vi "Test Menu Module API.vi"() -> ()   [LabVIEW 2019]
doc: "Menu Module API Tester."
uses:
  Utility/Controls/Menu_Configuration.ctl
  Menu Module.lvlib
panel:
  in  "Menu Type":enum16{"Root", "Sub", "Child"}(ring)
  out "selected Option":string
  in  "Position":cluster{"Top":i16, "Left":i16}
  in  "Resize the Panel":bool
  in  "Menu_Configuration":T1={"Button_Label_Color"=0, "Button_Color_On"=13762511, "Button_Color_Off"=13762511, "Panel_Color"=13762511, "Extend_Sub_Menu_Icon"=path "C:/Users/SyncSols-4/Desktop/Icon/add-icon.png", "Root_Menu_Data"=[{"Button_Icon"=path "C:/Users/SyncSols-4/Desktop/Icon/Accept-icon.png", "Button_Label"="Test", "Sub_Menu_Data"=[{"Button_Icon"=path "C:/Users/SyncSols-4/Desktop/Icon/floppy-icon.png", "Button_Label"="Save", "Child_Menu_Data"=[]}, {"Button_Icon"=path "C:/Users/SyncSols-4/Desktop/Icon/folder-icon1.png", "Button_Label"="Folder", "Child_Menu_Data"=[]}, {"Button_Icon"=path "C:/Users/SyncSols-4/Desktop/Icon/delete-icon.png", "Button_Label"="Delete", "Child_Menu_Data"=[{"Button_Icon"=path "C:/Users/SyncSols-4/Desktop/Icon/add-icon.png", "Button_Label"="Add"}, {"Button_Icon"=path "C:/Users/SyncSols-4/Desktop/Icon/Stop-red-icon.png", "Button_Label"="Stop"}]}]}, {"Button_Icon"=path "C:/Users/SyncSols-4/Desktop/Icon/add-key-icon.png", "Button_Label"="Key", "Sub_Menu_Data"=[]}, {"Button_Icon"=path "C:/Users/SyncSols-4/Desktop/Icon/Categories-preferences-system-icon.png", "Button_Label"="Setting", "Sub_Menu_Data"=[]}]}
  in  "Init Menu":bool
  in  "Run as Singleton?":bool
  in  "Show Block Diagram":bool
  in  "Refresh Modules":bool
  out "Active Modules":string[](array[string])
  in  "Stop Module":bool
  in  "Select Module":i32(ring)=-1 caption="Select Module\nTo send Request to" items=["All"=-1]
  in  "Run New Module":bool
  in  "Hide Module Panel":bool
  in  "Show Module Panel":bool
  out "Status":string
  # "This VI tests the API for the Module."
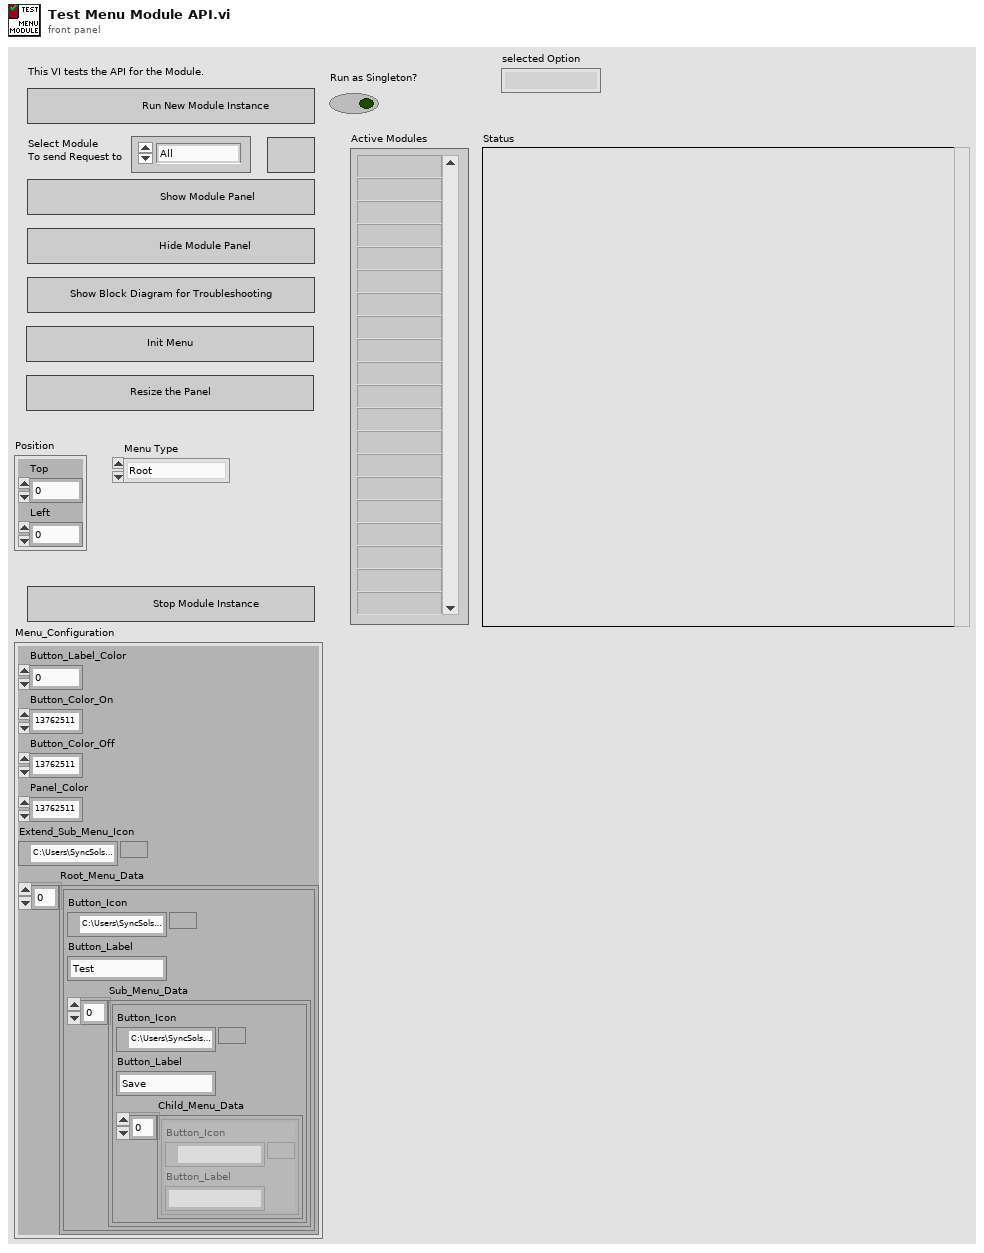
[diagram p1: front panel]
types:
  T1 = typedef "Menu_Configuration.ctl" = cluster{"Button_Label_Color":u32, "Button_Color_On":u32, "Button_Color_Off":u32, "Panel_Color":u32, "Extend_Sub_Menu_Icon":path, "Root_Menu_Data":cluster{"Button_Icon":path, "Button_Label":string, "Sub_Menu_Data":cluster{"Button_Icon":path, "Button_Label":string, "Child_Menu_Data":cluster{"Button_Icon":path, "Button_Label":string}[]}[]}[]}
  T2 = typedef "Menu Module.lvlib/Broadcast Events--cluster.ctl" = cluster{"Module Did Init":refnum<user-event>, "Status Updated":refnum<user-event>, "Error Reported":refnum<user-event>, "Module Did Stop":refnum<user-event>, "Update Module Execution Status":refnum<user-event>, "Button Pressed":refnum<user-event>}
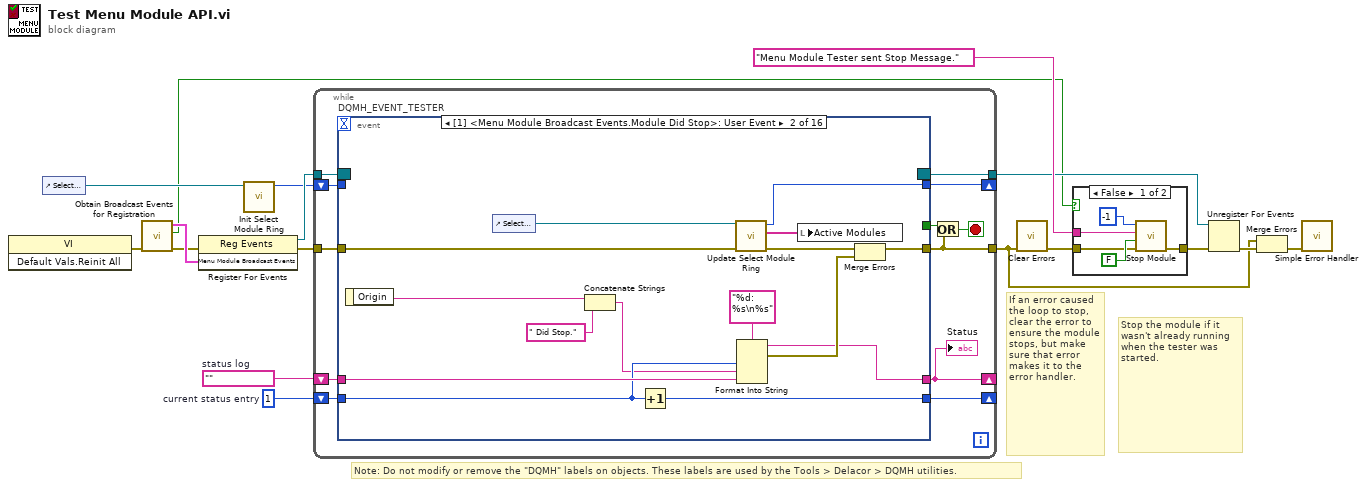
[diagram p0: block diagram]
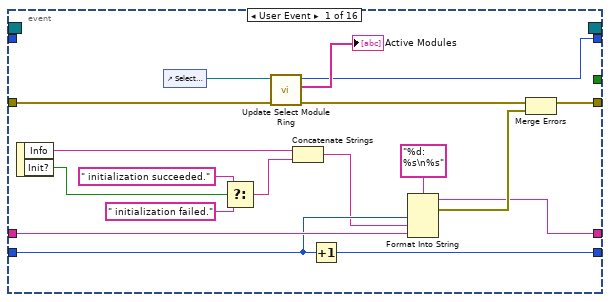
[diagram p3: hidden frame]
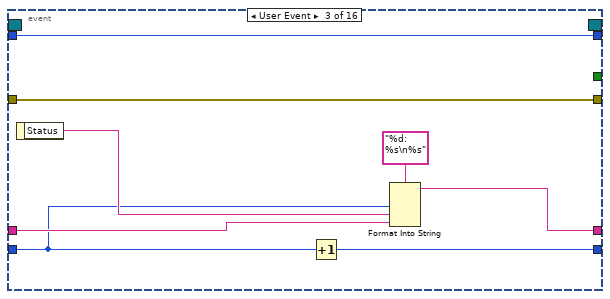
[diagram p4: hidden frame]
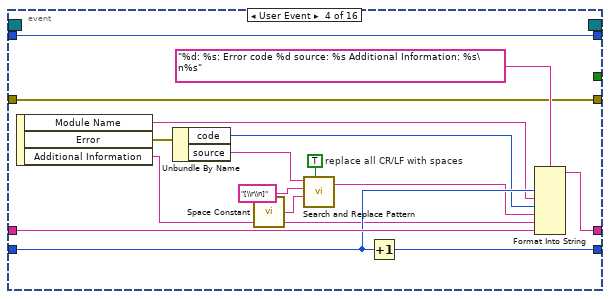
[diagram p5: hidden frame]
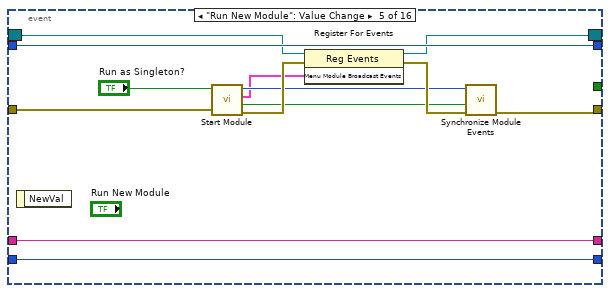
[diagram p6: hidden frame]
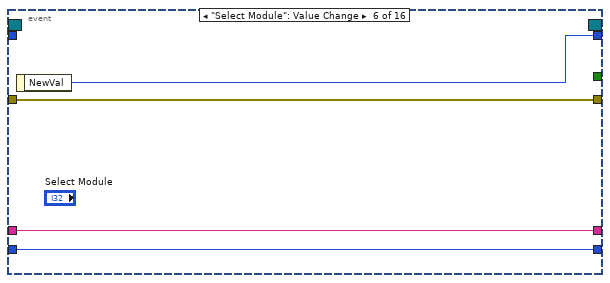
[diagram p7: hidden frame]
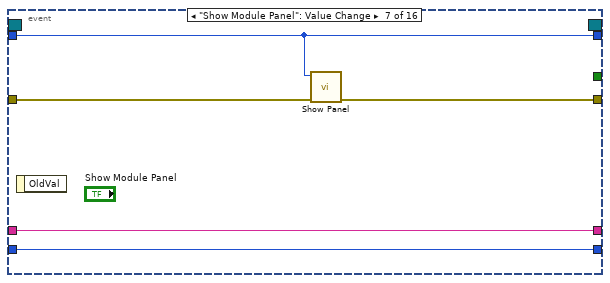
[diagram p8: hidden frame]
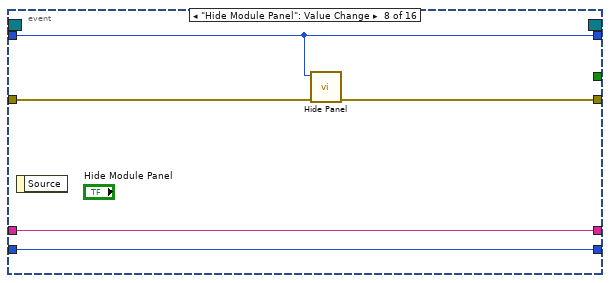
[diagram p9: hidden frame]
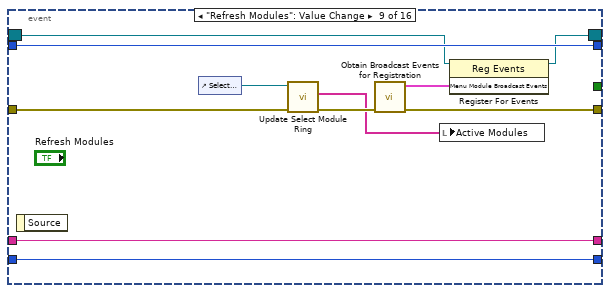
[diagram p10: hidden frame]
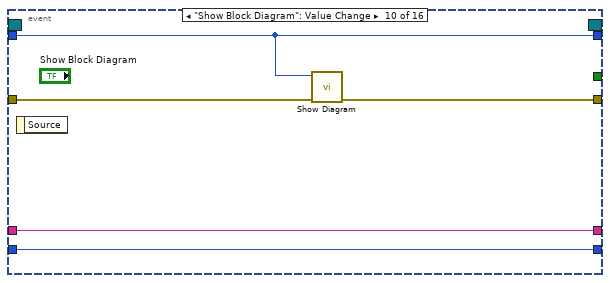
[diagram p11: hidden frame]
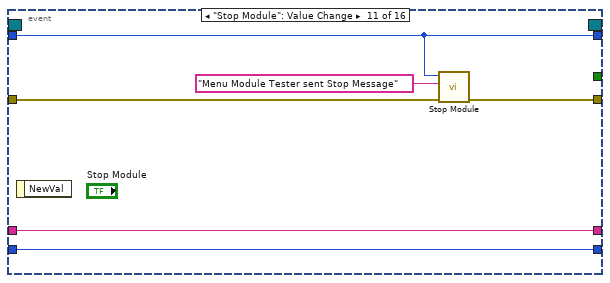
[diagram p12: hidden frame]
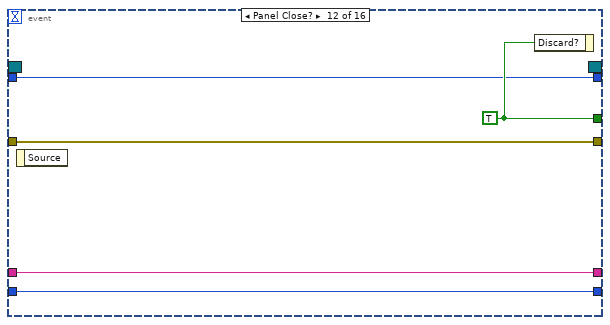
[diagram p13: hidden frame]
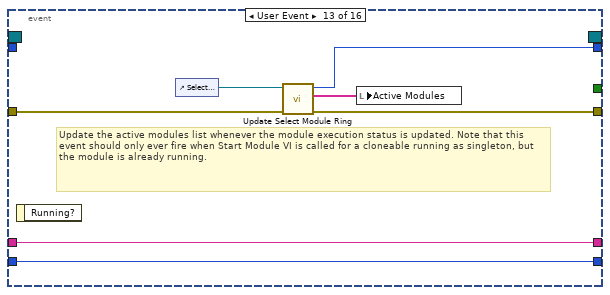
[diagram p14: hidden frame]
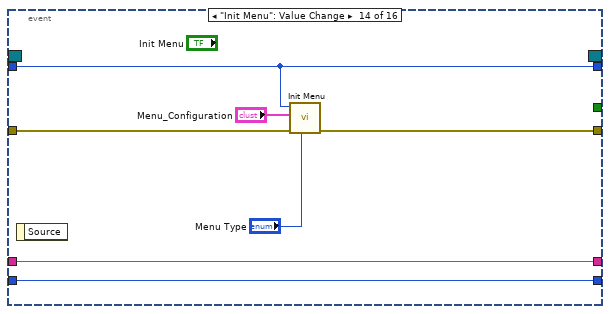
[diagram p15: hidden frame]
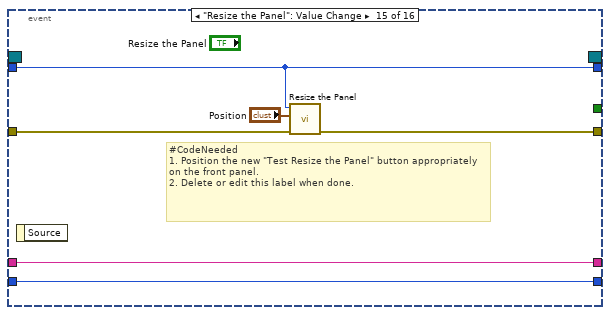
[diagram p16: hidden frame]
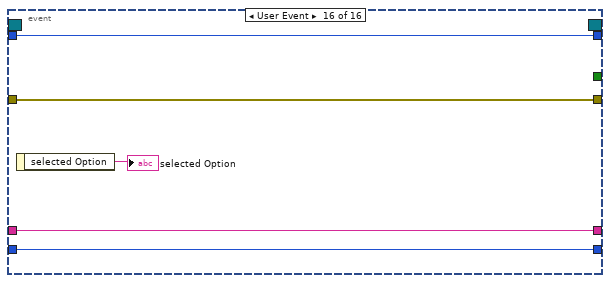
[diagram p17: hidden frame]
diagram:
  w13 = 1  # current status entry
  w14 = ""  # status log
  # "Stop the module if it wasn't already running when the tester was started."
  # "If an error caused the loop to stop, clear the error to ensure the module stops, but make sure that error makes it to the error handler."
  # "Note: Do not modify or remove the \"DQMH\" labels on objects. These labels are used by the Tools > Delacor > DQMH utilities."
  n1 = invoke class="VI" method="Default Vals.Reinit All"() -> (error out=w3:errorcluster)  [unwired: 3 in, 2 out]
  n2 = control-ref of="Select Module"() -> (w11:refnum<vi>)
  n3 = call "Obtain Broadcast Events for Registration.vi"("error in (no error)"=w3) -> ("error out"=w2:errorcluster, "Already running?"=w1:bool, "Menu Module Broadcast Events"=w10:T2)  [unwired: 8 in]
  n4 = register-events(error in=w2, w10) -> (reference out=w17:refnum<event-registration>, error out=w9:errorcluster)  [unwired: 1 in]
  n5 = call "Init Select Module Ring.vi"("Select Module Ring Ref"=w11) -> ("Value for All Modules"=w12:i32)  [unwired: 8 in, 2 out]
  n6 = while {
    tunnel: w17 -> [w29]
    tunnel: [w18] -> w4
    tunnel: w9 -> [w27]
    shift-right: [w23] -> _
    shift-left: w14 -> [w25]
    shift-right: [w24] -> _
    shift-left: w13 -> [w26]
    shift-right: [w20] -> _
    shift-left: w12 -> [w21]
    tunnel: [w19] -> w7
    stop <- w22 stop-if-true
    n7 = event "DQMH_EVENT_TESTER" shown="[1] <Menu Module Broadcast Events.Module Did Stop>: User Event" {
      selector: w29 -> [_ _ _ _ w93 _ _ _ w119 _ _ _ _ _ _ _]
      dyn-events: [_ _ _ _ w92 _ _ _ w118 _ _ _ _ _ _ _] -> w19
      timeout: _ -> [_ _ _ _ _ _ _ _ _ _ _ _ _ _ _ _]
      tunnel: [_ _ _ _ _ _ _ _ _ _ _ w140 _ _ _ _] -> w28
      tunnel: [w37 w54 w70 w76 w91 w103 w107 w112 w115 w126 w131 w139 w143 w151 w157 w165] -> w18
      tunnel: w27 -> [w39 w56 w70 w76 w94 w103 w108 w113 w120 w129 w132 w139 w144 w154 w160 w165]
      tunnel: w26 -> [w44 w59 w63 w82 w96 w101 w105 w110 w123 w127 w134 w137 w146 w152 w158 w163]
      tunnel: w25 -> [w45 w60 w66 w84 w97 w102 w106 w111 w124 w128 w135 w138 w147 w153 w159 w164]
      tunnel: [w42 w57 w67 w79 w97 w102 w106 w111 w124 w128 w135 w138 w147 w153 w159 w164] -> w23
      tunnel: [w43 w58 w69 w85 w96 w101 w105 w110 w123 w127 w134 w137 w146 w152 w158 w163] -> w24
      tunnel: w21 -> [_ _ w64 w86 w95 _ w104 w109 w122 w125 w133 w136 _ w150 w156 w162]
      tunnel: [w34 w51 w64 w86 w95 w100 w104 w109 w122 w125 w133 w136 w142 w150 w156 w162] -> w20
      event User Event {
        n8 = event-data() -> ("Info"=w41:string, "Init?"=w31:bool)  [unwired: 1 in]
        n9 = control-ref of="Select Module"() -> (w36:refnum<vi>)
        n10 = Select(t=" initialization succeeded.", s=w31, f=" initialization failed.") -> (s? t:f=w30:string)
        n11 = call "Update Select Module Ring.vi"("error in (no error)"=w39, "Select Module Ring Ref"=w36) -> ("error out"=w38:errorcluster, "Active Modules (Array)"=→"Active Modules":string[], "New Module Ring Value"=w34:i32)  [unwired: 7 in]
        n12 = Concatenate Strings(w41, w30) -> (w40:string)
        n13 = Increment(x=w44) -> (x+1=w43:i32)
        n14 = Format Into String(format string="%d: %s\n%s", w44, w40, w45) -> (resulting string=w42:string, error out=w47:errorcluster)  [unwired: 2 in]
        n15 = Merge Errors(w38, w47) -> (w37:errorcluster)
      }
      event User Event {
        n16 = event-data() -> ("Origin"=w49:string)  [unwired: 1 in]
        n17 = control-ref of="Select Module"() -> (w53:refnum<vi>)
        n18 = Concatenate Strings(w49, " Did Stop.") -> (w48:string)
        n19 = Increment(x=w59) -> (x+1=w58:i32)
        n20 = call "Update Select Module Ring.vi"("error in (no error)"=w56, "Select Module Ring Ref"=w53) -> ("error out"=w55:errorcluster, "Active Modules (Array)"=w52:string[], "New Module Ring Value"=w51:i32)  [unwired: 7 in]
        n21 = Format Into String(format string="%d: %s\n%s", w59, w48, w60) -> (resulting string=w57:string, error out=w62:errorcluster)  [unwired: 2 in]
        n22 = local write "Active Modules"(w52) -> ()
        n23 = Merge Errors(w55, w62) -> (w54:errorcluster)
      }
      event User Event {
        n24 = event-data() -> ("Status"=w65:string)  [unwired: 1 in]
        n25 = Increment(x=w63) -> (x+1=w69:i32)
        n26 = Format Into String(format string="%d: %s\n%s", w63, w65, w66) -> (resulting string=w67:string)  [unwired: 2 in, 1 out]
      }
      event User Event {
        w80 = TRUE  # replace all CR/LF with spaces
        n27 = event-data() -> ("Module Name"=w74:string, "Error"=w73:errorcluster, "Additional Information"=w71:string)  [unwired: 1 in]
        n28 = Unbundle By Name(w73) -> ("code"=w75:i32, "source"=w77:string)
        n29 = call <vilib>:"Space Constant.vi"() -> ("String"=w81:string)
        n30 = call <vilib>:"Search and Replace Pattern.vi"("string"=w77, "regular expression (\"\")"="[\\r\\n]" ("regular expression (\"\")"), "replace string (\"\")"=w81, "replace all? (F)"=w80) -> ("result string"=w78:string)  [unwired: 1 in, 1 out]
        n31 = Increment(x=w82) -> (x+1=w85:i32)
        n32 = Format Into String(format string="%d: %s: Error code %d source: %s Additional Information: %s\n%s", w82, w74, w75, w78, w71, w84) -> (resulting string=w79:string)  [unwired: 2 in, 1 out]
      }
      event "Run New Module": Value Change {
        n33 = event-data() -> ()  [unwired: 1 in, 1 out]
        n34 = call "Start Module.vi"("error in (no error)"=w94, "Run as Singleton? (F)"="Run as Singleton?") -> ("error out"=w98:errorcluster, "Wait for Event Sync?"=w89:bool, "Menu Module Broadcast Events"=w88:T2, "Module ID"=w90:i32)  [unwired: 6 in]
        n35 = register-events(reference=w93, error in=w98, w88) -> (reference out=w92:refnum<event-registration>, error out=w99:errorcluster)
        n36 = call "Synchronize Module Events.vi"("error in (no error)"=w99, "Wait for Event Sync?"=w89, "Module ID"=w90) -> ("error out"=w91:errorcluster)  [unwired: 7 in, 1 out]
      }
      event "Select Module": Value Change {
        n37 = event-data() -> ("NewVal"=w100:i32)  [unwired: 1 in]
      }
      event "Show Module Panel": Value Change {
        n38 = event-data() -> ()  [unwired: 1 in, 1 out]
        n39 = call "Show Panel.vi"("error in (no error)"=w108, "Module ID"=w104) -> ("error out"=w107:errorcluster)  [unwired: 9 in]
      }
      event "Hide Module Panel": Value Change {
        n40 = event-data() -> ()  [unwired: 1 in, 1 out]
        n41 = call "Hide Panel.vi"("error in (no error)"=w113, "Module ID"=w109) -> ("error out"=w112:errorcluster)  [unwired: 9 in]
      }
      event "Refresh Modules": Value Change {
        n42 = event-data() -> ()  [unwired: 1 in, 1 out]
        n43 = control-ref of="Select Module"() -> (w121:refnum<vi>)
        n44 = call "Update Select Module Ring.vi"("error in (no error)"=w120, "Select Module Ring Ref"=w121) -> ("error out"=w116:errorcluster, "Active Modules (Array)"=w114:string[])  [unwired: 7 in, 1 out]
        n45 = call "Obtain Broadcast Events for Registration.vi"("error in (no error)"=w116) -> ("error out"=w115:errorcluster, "Menu Module Broadcast Events"=w117:T2)  [unwired: 8 in, 1 out]
        n46 = local write "Active Modules"(w114) -> ()
        n47 = register-events(reference=w119, w117) -> (reference out=w118:refnum<event-registration>)  [unwired: 1 in, 1 out]
      }
      event "Show Block Diagram": Value Change {
        n48 = event-data() -> ()  [unwired: 1 in, 1 out]
        n49 = call "Show Diagram.vi"("error in (no error)"=w129, "Module ID"=w125) -> ("error out"=w126:errorcluster)  [unwired: 9 in]
      }
      event "Stop Module": Value Change {
        n50 = event-data() -> ()  [unwired: 1 in, 1 out]
        n51 = call "Stop Module.vi"("error in (no error)"=w132, "Origin"="Menu Module Tester sent Stop Message", "Module ID"=w133) -> ("error out"=w131:errorcluster)  [unwired: 8 in]
      }
      event Panel Close? {
        w140 = TRUE ("Discard?")
        n52 = event-data() -> ()  [unwired: 1 in, 1 out]
        n53 = event-data("Discard?"=w140) -> ()  [unwired: 1 in, 1 out]
      }
      event User Event {
        # "Update the active modules list whenever the module execution status is updated. Note that this event should only ever fire when Start Module VI is called for a cloneable running as singleton, but the module is already running."
        n54 = event-data() -> ()  [unwired: 1 in, 1 out]
        n55 = control-ref of="Select Module"() -> (w145:refnum<vi>)
        n56 = call "Update Select Module Ring.vi"("error in (no error)"=w144, "Select Module Ring Ref"=w145) -> ("error out"=w143:errorcluster, "Active Modules (Array)"=w141:string[], "New Module Ring Value"=w142:i32)  [unwired: 7 in]
        n57 = local write "Active Modules"(w141) -> ()
      }
      event "Init Menu": Value Change {
        n58 = event-data() -> ()  [unwired: 1 in, 1 out]
        n59 = call "Init Menu.vi"("Menu Type"="Menu Type", "error in (no error)"=w154, "Menu_Configuration"="Menu_Configuration", "Module ID"=w150) -> ("error out"=w151:errorcluster)  [unwired: 7 in]
      }
      event "Resize the Panel": Value Change {
        # "#CodeNeeded\n1. Position the new \"Test Resize the Panel\" button appropriately on the front panel.\n2. Delete or edit this label when done."
        n60 = event-data() -> ()  [unwired: 1 in, 1 out]
        n61 = call "Resize the Panel.vi"("error in (no error)"=w160, "Position"="Position", "Module ID"=w156) -> ("error out"=w157:errorcluster)  [unwired: 8 in]
      }
      event User Event {
        n62 = event-data() -> ("selected Option"=→"selected Option":string)  [unwired: 1 in]
      }
    }
    "Status" <- w23
    n63 = Or(x=w28, y=w18) -> (x .or. y?=w22:bool)
  }
  n64 = call <vilib>:"Clear Errors.vi"("error in (no error)"=w4) -> ("error out"=w6:errorcluster)  [unwired: 5 in, 1 out]
  n65 = case shown="False" w1 {
    tunnel: [w170 w171] -> w15
    tunnel: "Menu Module Tester sent Stop Message." ("Origin") -> [w169 _]
    tunnel: w6 -> [w166 w171]
    frame False {
      n66 = call "Stop Module.vi"("error in (no error)"=w166, "Wait for Module to stop? (F)"=FALSE ("Wait for Module to stop?"), "Origin"=w169, "Module ID"=-1 ("Stop all")) -> ("error out"=w170:errorcluster)  [unwired: 7 in]
    }
    frame True {
    }
  }
  n67 = Unregister For Events(event registration refnum=w7, error in=w15) -> (error out=w16:errorcluster)
  n68 = Merge Errors(w4, w16) -> (w5:errorcluster)
  n69 = call <vilib>:"Simple Error Handler.vi"("error in (no error)"=w5) -> ()  [unwired: 4 in, 5 out]
